vi "APC_isOk.vi"(8 "error in (no error)":errorcluster) -> (0 "error out":errorcluster, 3 "Power OK?":bool)   [LabVIEW 2018]
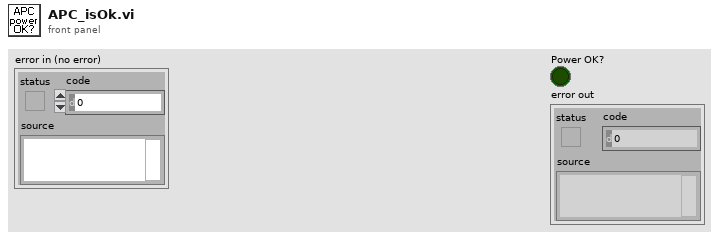
[diagram p1: front panel]
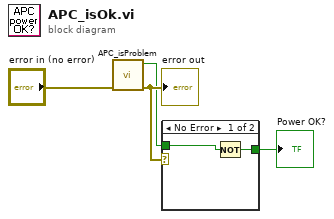
[diagram p0: block diagram]
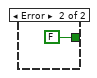
[diagram p2: hidden frame]
diagram:
  n1 = call "APC_isProblem.vi"("error in (no error)"="error in (no error)") -> ("error out"=w3:errorcluster, "PowerProblem?"=w2:bool)  [unwired: 9 in]
  "error out" <- w3
  n2 = case shown="No Error" w3 {
    tunnel: w2 -> [w6 _]
    tunnel: [w5 FALSE] -> w1
    frame No Error {
      n3 = Not(x=w6) -> (.not. x?=w5:bool)
    }
    frame Error {
    }
  }
  "Power OK?" <- w1
